vi "Handle Command.vi"(8 "error in (no error)":errorcluster, 10 "CMD in":refnum<class "Change Speaker Switch State.lvclass">, 11 "Object In":refnum<class>) -> (0 "error out":errorcluster, 1 "Command Successful?":bool, 2 "CMD out":refnum<class "Change Speaker Switch State.lvclass">, 3 "Object Out":refnum<class>)   [LabVIEW 2014, in "ePAS Library.lvlib" / "Change Speaker Switch State.lvclass"]
uses:
  Change Speaker Switch State.lvclass
  reusable/PAS/Main/PAS.lvclass
  reusable/Instrument/Instrument.lvclass/Instrument.ctl
  Change Speaker Switch State.lvclass/Change Speaker Switch State.ctl
  reusable/Switch/Switch.lvclass/Switch.ctl
  reusable/Instrument/Read ExtCom.vi
  reusable/Instrument/Read Log Session.vi
  reusable/Switch/Write Cycle_.vi
  reusable/PAS/Main/Read Switch Ref.vi
  reusable/Switch/Write maxElapseTime.vi
  reusable/PAS/Main/Write Speaker Reference.vi
  reusable/Switch/Switch.lvclass
  <userlib>/_Session Fwk/Session - Root.lvclass
  reusable/Session APIs/Session Log/System Log.lvclass
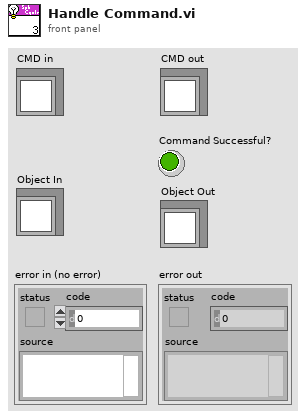
[diagram p1: front panel]
types:
  T1 = typedef "Session - Root.lvclass/Session Handle.ctl" = refnum<data-value>
  T2 = cluster{"tag":string, "section":string, "data":variant}
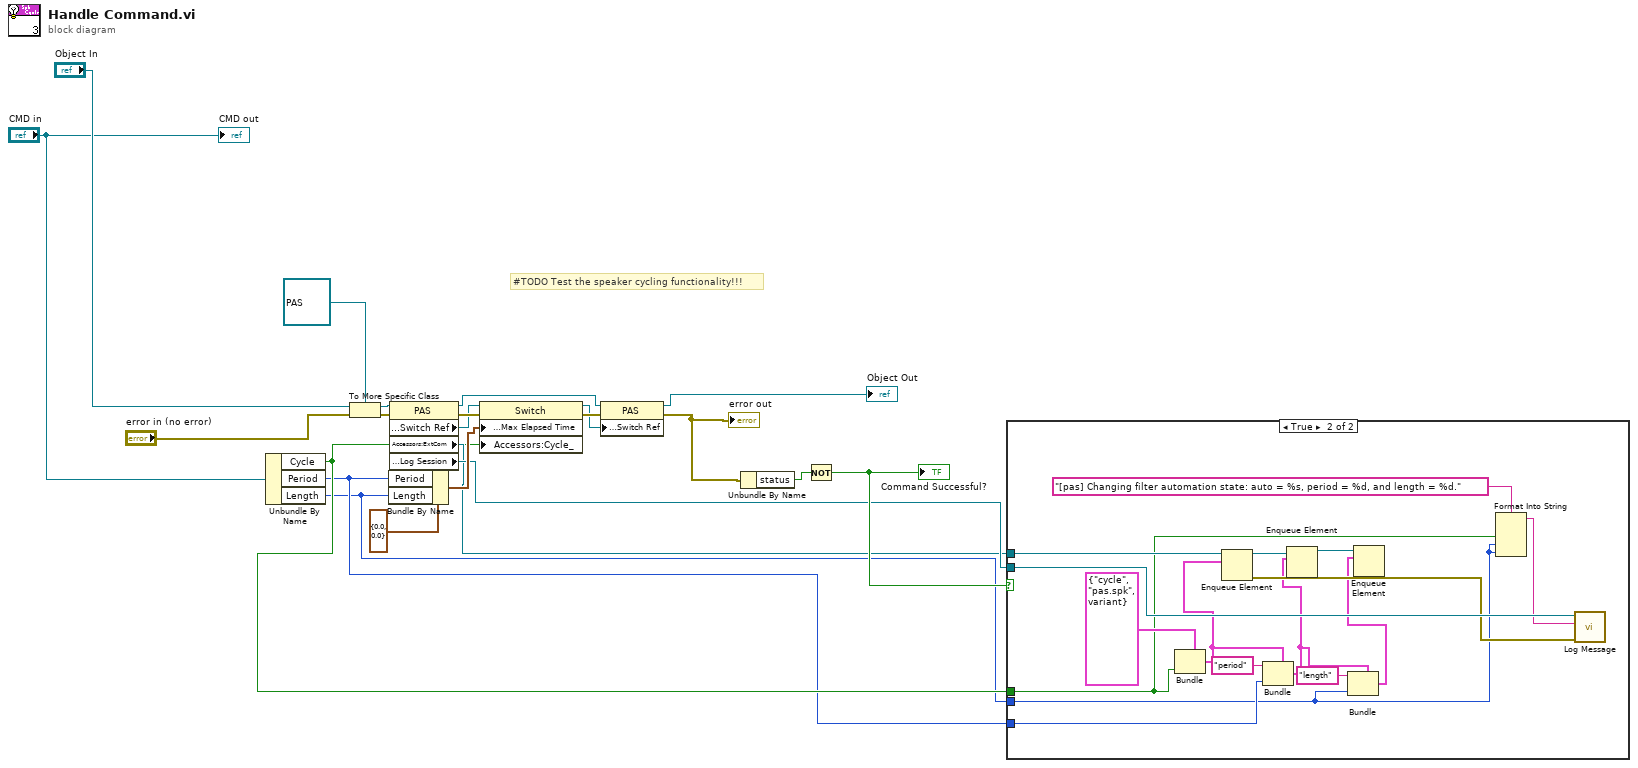
[diagram p0: block diagram]
diagram:
  # "#TODO Test the speaker cycling functionality!!!"
  n1 = Unbundle By Name("CMD in") -> ("Cycle"=w3:bool, "Period"=w2:i16, "Length"=w1:i16)
  n2 = To More Specific Class(target class=refnum<class "PAS.lvclass"> refnum ("PAS"), reference="Object In", error in="error in (no error)") -> (specific class reference=w22:refnum<class "PAS.lvclass">, error out=w20:errorcluster)
  n3 = Bundle By Name(cluster=cluster{"Period":sgl, "Length":sgl} {"Period"=0.0, "Length"=0.0} ("Max Elapsed Time"), "Period"=w2, "Length"=w1) -> (w13:cluster{"Period":sgl, "Length":sgl})
  n4 = property class="PAS"(reference=w22, error in=w20) -> (reference out=w17:refnum<class "PAS.lvclass">, error out=w21:errorcluster, "Data Access:Switch Ref"=w18:refnum<class "Switch.lvclass">, "Accessors:ExtCom"=w4:refnum<queue>, "Accessors:Log Session"=w5:T1)
  n5 = property class="Switch"(reference=w18, error in=w21, "Data Access:Max Elapsed Time"=w13, "Accessors:Cycle_"=w3) -> (reference out=w15:refnum<class "Switch.lvclass">, error out=w16:errorcluster)
  n6 = property class="PAS"(reference=w17, error in=w16, "Data Access:Switch Ref"=w15) -> (reference out=→"Object Out":refnum<class "PAS.lvclass">, error out=w7:errorcluster)
  "error out" <- w7
  n7 = Unbundle By Name(w7) -> ("status"=w8:bool)
  n8 = Not(x=w8) -> (.not. x?=w6:bool)
  "Command Successful?" <- w6
  n9 = case shown="True" w6 {
    tunnel: w4 -> [_ w38]
    tunnel: w5 -> [_ w36]
    tunnel: w3 -> [_ w25]
    tunnel: w2 -> [_ w27]
    tunnel: w1 -> [_ w24]
    frame False {
    }
    frame True {
      n10 = Bundle(cluster=T2 {"tag"="cycle", "section"="pas.spk", "data"=variant} ("element"), "data"=w25) -> (w32:T2)  [unwired: 2 in]
      n11 = Enqueue Element(queue=w38, element=w32) -> (queue out=w34:refnum<queue>, error out=w35:errorcluster)  [unwired: 2 in, 1 out]
      n12 = Bundle(cluster=w32, "tag"="period", "data"=w27) -> (w30:T2)  [unwired: 1 in]
      n13 = Enqueue Element(queue=w34, element=w30) -> (queue out=w33:refnum<queue>)  [unwired: 2 in, 2 out]
      n14 = Bundle(cluster=w30, "tag"="length", "data"=w24) -> (w28:T2)  [unwired: 1 in]
      n15 = Enqueue Element(queue=w33, element=w28) -> ()  [unwired: 2 in, 3 out]
      n16 = Format Into String(format string="[pas] Changing filter automation state: auto = %s, period = %d, and length = %d.", w25, w24, w24) -> (resulting string=w23:string)  [unwired: 2 in, 1 out]
      n17 = call "Log Message.vi"("error in"=w35, "MSG In"=w23, "session in"=w36) -> ()  [unwired: 7 in, 2 out]
    }
  }
  "CMD out" <- "CMD in"
